vi "hmi_load_project.vi"(7 "hmi_references":T2, 8 "error in (no error)":errorcluster, 9 "commit_hash":string, 10 "config":T1, 11 "build_spec []":T3[](array[typedef])) -> (0 "error out":errorcluster)   [LabVIEW 2015, in "lv-build-interface.lvlib"]
uses:
  lv-build-interface.lvlib
  lv-build/public/_controls/build_specification.ctl
  lv-build/public/_controls/build_type.ctl
  _controls/hmi_references.ctl
  lv-build/public/_controls/configuration.ctl
  lv-builder/class/lv-builder.lvclass
  lv-build/lv-build.lvlib
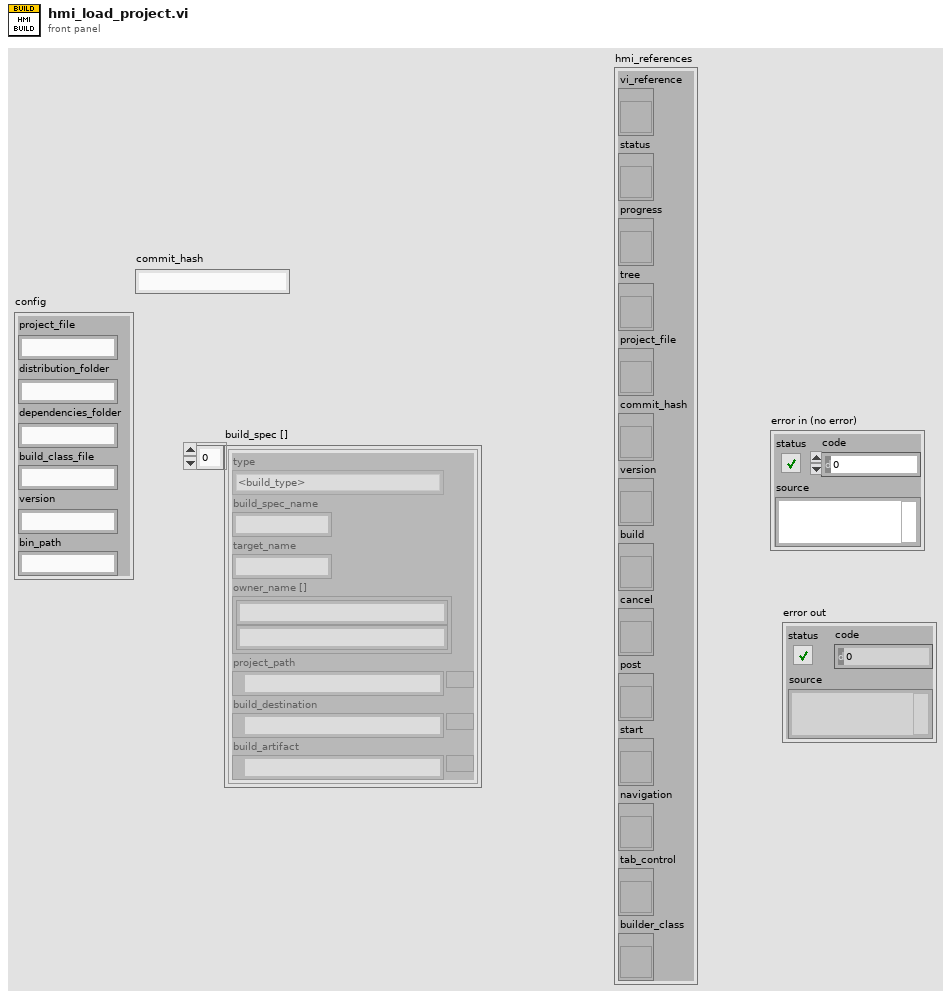
[diagram p1: front panel]
types:
  T1 = typedef "lv-build.lvlib/configuration.ctl" = cluster{"project_file":string, "distribution_folder":string, "dependencies_folder":string, "build_class_file":string, "version":string, "bin_path":string}
  T2 = typedef "lv-build-interface.lvlib/hmi_references.ctl" = cluster{"vi_reference":refnum<vi>, "status":refnum<vi>, "progress":refnum<vi>, "tree":refnum<vi>, "project_file":refnum<vi>, "commit_hash":refnum<vi>, "version":refnum<vi>, "build":refnum<vi>, "cancel":refnum<vi>, "post":refnum<vi>, "start":refnum<vi>, "navigation":refnum<vi>, "tab_control":refnum<vi>, "builder_class":refnum<vi>}
  T3 = typedef "lv-build.lvlib/build_specification.ctl" = cluster{"type":T4, "build_spec_name":string, "target_name":string, "owner_name []":string[], "project_path":path, "build_destination":path, "build_artifact":path}
  T4 = typedef "lv-build.lvlib/build_type.ctl" = enum16{"<build_type>", "application_pc", "application_rt", "installer", "llb", "lvlibp", "zip", "fpga", "<null>"}
  T5 = cluster{cluster{"build_spec_name":string, i32}[]}
  T6 = cluster{"target_name":string, "build_spec_name":string, i32}
  T7 = cluster{"target_name":string, "build_spec_name":string, i32}[]
  T8 = cluster{cluster{"build_spec_name":string, i32}[]}[]
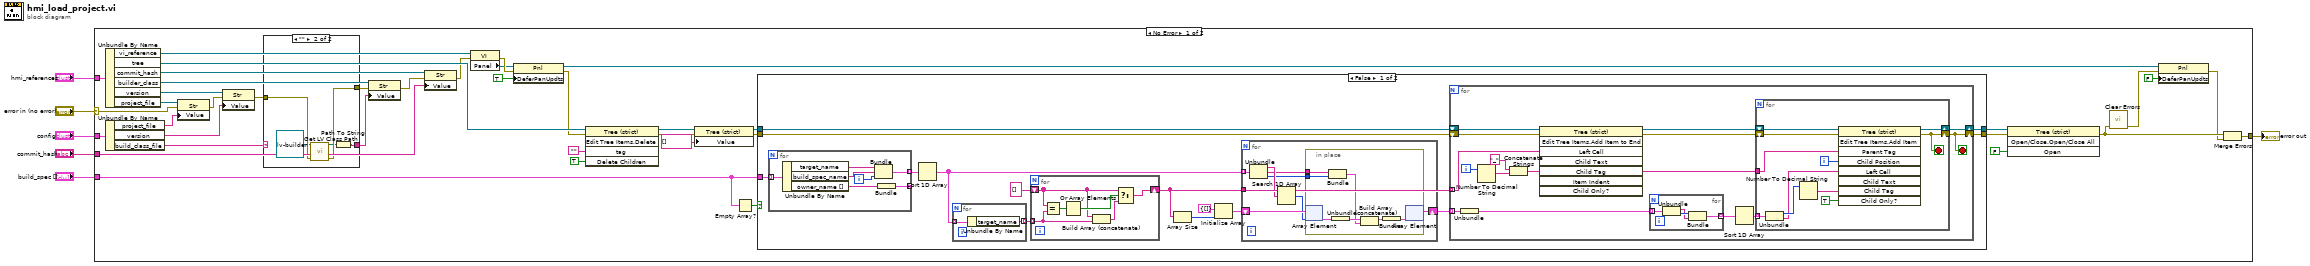
[diagram p0: block diagram]
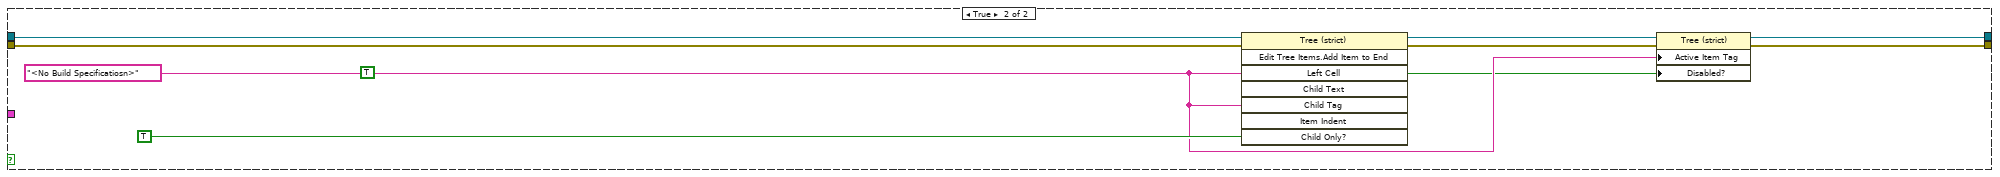
[diagram p3: hidden frame]
diagram:
  n1 = case shown="No Error" "error in (no error)" {
    selector: "error in (no error)" -> [w26 w138]
    tunnel: "hmi_references" -> [w47 _]
    tunnel: "config" -> [w18 _]
    tunnel: "build_spec []" -> [w30 _]
    tunnel: [w20 w138] -> w3
    tunnel: "commit_hash" -> [w15 _]
    frame No Error {
      n2 = Unbundle By Name(w47) -> ("vi_reference"=w27:refnum<vi>, "tree"=w29:refnum<vi>, "commit_hash"=w24:refnum<vi>, "builder_class"=w12:refnum<vi>, "version"=w17:refnum<vi>, "project_file"=w28:refnum<vi>)
      n3 = Unbundle By Name(w18) -> ("project_file"=w13:string, "version"=w14:string, "build_class_file"=w10:string)
      n4 = property class="Str"(reference=w28, error in=w26, "Value"=w13) -> (error out=w16:errorcluster)  [unwired: 1 out]
      n5 = property class="Str"(reference=w17, error in=w16, "Value"=w14) -> (error out=w9:errorcluster)  [unwired: 1 out]
      n6 = case shown="\"\"" w10 {
        selector: w10 -> [w49 _]
        tunnel: w9 -> [w48 w54]
        tunnel: [w49 w50] -> w8
        tunnel: [w48 w52] -> w7
        frame Default {
        }
        frame "" {
          n7 = call <vilib>:"Get LV Class Path.vi"("error in (no error)"=w54, "object"=refnum<class "lv-builder.lvclass"> refnum ("lv-builder.lvlib:lv-builder.lvclass")) -> ("error out"=w52:errorcluster, "class path"=w51:path)  [unwired: 8 in]
          n8 = Path To String(path=w51) -> (string=w50:string)
        }
      }
      n9 = property class="Str"(reference=w12, error in=w7, "Value"=w8) -> (error out=w11:errorcluster)  [unwired: 1 out]
      n10 = property class="Str"(reference=w24, error in=w11, "Value"=w15) -> (error out=w23:errorcluster)  [unwired: 1 out]
      n11 = property class="VI"(reference=w27, error in=w23) -> (error out=w46:errorcluster, "Panel"=w45:refnum<vi>)  [unwired: 1 out]
      n12 = property class="Pnl"(reference=w45, error in=w46, "DeferPanUpdts"=TRUE ("Defer Panel Updates")) -> (reference out=w42:refnum<vi>, error out=w25:errorcluster)
      n13 = invoke class="Tree (strict)" method="Edit Tree Items.Delete"(reference=w29, error in=w25, "tag"="", "Delete Children"=TRUE ("Delete Children?")) -> (reference out=w34:refnum<vi>, error out=w33:errorcluster)  [unwired: 1 in, 3 out]
      n14 = property class="Tree (strict)"(reference=w34, error in=w33, "Value"=string[] []) -> (reference out=w36:refnum<vi>, error out=w35:errorcluster)
      n15 = Empty Array?(array=w30) -> (empty?=w32:bool)
      n16 = case shown="False" w32 {
        tunnel: [w68 w133] -> w38
        tunnel: [w67 w132] -> w37
        tunnel: w36 -> [w66 w136]
        tunnel: w35 -> [w65 w135]
        tunnel: w30 -> [w64 _]
        frame False {
          n17 = for {
            tunnel: [w81] -> w63 mode=indexing
            tunnel: w64 -> [w80] mode=indexing
            tunnel: [w77] -> _ mode=indexing
            i -> [w79]
            n18 = Unbundle By Name(w80) -> ("target_name"=w83:string, "build_spec_name"=w82:string, "owner_name []"=w78:string[])
            n19 = Bundle("target_name"=w83, "build_spec_name"=w82, w79) -> (w81:T6)  [unwired: 1 in]
            n20 = Bundle("owner_name []"=w78) -> (w77:cluster{"owner_name []":string[]})  [unwired: 1 in]
          }
          n21 = Sort 1D Array(array=w63) -> (sorted array=w59:T7)
          n22 = for {
            tunnel: w59 -> [w76] mode=indexing
            tunnel: [w75] -> w56 mode=indexing
            n23 = Unbundle By Name(w76) -> ("target_name"=w75:string)
          }
          n24 = for {
            shift-right: [w69] -> w55
            shift-left: string[] [] -> [w71]
            tunnel: w56 -> [w73] mode=indexing
            n25 = Equal?(x=w71, y=w73) -> (x = y?=w74:bool[])
            n26 = Or Array Elements(Boolean array=w74) -> (logical OR=w72:bool)
            n27 = Build Array (concatenate)(w71, w73) -> (w70:string[])
            n28 = Select(t=w71, s=w72, f=w70) -> (s? t:f=w69:string[])
          }
          n29 = Array Size(array=w55) -> (size(s)=w61:i32)
          n30 = Initialize Array(T5 {[]}, w61) -> (w60:T8)
          n31 = for {
            shift-right: [w87] -> w58
            shift-left: w60 -> [w89]
            tunnel: w59 -> [w91] mode=indexing
            tunnel: w55 -> [w90]
            n32 = Unbundle(w91) -> ("target_name"=w86:string, "build_spec_name"=w85:string, w84:i32)
            n33 = Search 1D Array(1D array=w90, element=w86) -> (index of element=w88:i32)  [unwired: 1 in]
            n34 = in-place {
              in-place-border: w85 -> [w94]
              in-place-border: w84 -> [w93]
              n35 = in-place-array #1(w89, w88) -> (w98:T5)
              n36 = Bundle("build_spec_name"=w94, w93) -> (w92:cluster{"build_spec_name":string, i32})  [unwired: 1 in]
              n37 = Unbundle(w98) -> (w97:cluster{"build_spec_name":string, i32}[])
              n38 = Build Array (concatenate)(w97, w92) -> (w95:cluster{"build_spec_name":string, i32}[])
              n39 = Bundle(w95) -> (w96:T5)  [unwired: 1 in]
              n40 = in-place-array #1(w96) -> (w87:T8)  [unwired: 1 out]
            }
          }
          n41 = for {
            shift-right: [w109] -> w68
            shift-left: w66 -> [w113]
            shift-right: [w105] -> w67
            shift-left: w65 -> [w112]
            tunnel: w55 -> [w107] mode=indexing
            tunnel: w58 -> [w106] mode=indexing
            i -> [w108]
            stop <- w105 stop-if-true
            n42 = Unbundle(w106) -> (w101:cluster{"build_spec_name":string, i32}[])
            n43 = Number To Decimal String(number=w108) -> (decimal integer string=w103:string)  [unwired: 1 in]
            n44 = Concatenate Strings("_" ("string"), w103) -> (w102:string)
            n45 = invoke class="Tree (strict)" method="Edit Tree Items.Add Item to End"(reference=w113, error in=w112, "Left Cell"=w107, "Child Tag"=w102) -> (reference out=w111:refnum<vi>, error out=w110:errorcluster)  [unwired: 4 in, 6 out]
            n46 = for {
              tunnel: w101 -> [w117] mode=indexing
              tunnel: [w114] -> w100 mode=indexing
              n47 = Unbundle(w117) -> ("build_spec_name"=w115:string, w116:i32)
              n48 = Bundle(w116, "build_spec_name"=w115) -> (w114:cluster{i32, "build_spec_name":string})  [unwired: 1 in]
            }
            n49 = Sort 1D Array(array=w100) -> (sorted array=w99:cluster{i32, "build_spec_name":string}[])
            n50 = for {
              tunnel: w102 -> [w124]
              shift-right: [w126] -> w109
              shift-left: w111 -> [w128]
              shift-right: [w122] -> w105
              shift-left: w110 -> [w127]
              tunnel: w99 -> [w123] mode=indexing
              i -> [w121]
              stop <- w122 stop-if-true
              n51 = Unbundle(w123) -> (w119:i32, "build_spec_name"=w118:string)
              n52 = Number To Decimal String(number=w119) -> (decimal integer string=w120:string)  [unwired: 1 in]
              n53 = invoke class="Tree (strict)" method="Edit Tree Items.Add Item"(reference=w128, error in=w127, "Parent Tag"=w124, "Child Position"=w121, "Left Cell"=w118, "Child Tag"=w120, "Child Only?"=TRUE) -> (reference out=w126:refnum<vi>, error out=w122:errorcluster)  [unwired: 2 in, 7 out]
            }
          }
        }
        frame True {
          w130 = "<No Build Specificatiosn>"
          n54 = invoke class="Tree (strict)" method="Edit Tree Items.Add Item to End"(reference=w136, error in=w135, "Left Cell"=w130, "Child Tag"=w130, "Child Only?"=TRUE) -> (reference out=w134:refnum<vi>, error out=w131:errorcluster)  [unwired: 3 in, 6 out]
          n55 = property class="Tree (strict)"(reference=w134, error in=w131, "Active Item Tag"=w130, "Disabled?"=TRUE ("Active Item:Disabled?")) -> (reference out=w133:refnum<vi>, error out=w132:errorcluster)
        }
      }
      n56 = invoke class="Tree (strict)" method="Open/Close.Open/Close All"(reference=w38, error in=w37, "Open"=FALSE ("Open?")) -> (error out=w22:errorcluster)  [unwired: 1 in, 3 out]
      n57 = call <vilib>:"Clear Errors.vi"("error in (no error)"=w22) -> ("error out"=w19:errorcluster)  [unwired: 5 in, 1 out]
      n58 = property class="Pnl"(reference=w42, error in=w19, "DeferPanUpdts"=FALSE ("Defer Panel Updates")) -> (error out=w21:errorcluster)  [unwired: 1 out]
      n59 = Merge Errors(w22, w21) -> (w20:errorcluster)
    }
    frame Error {
    }
  }
  "error out" <- w3
